vi "SeqListBox_EditMode.vi"(8 "error in (no error)":errorcluster, 10 "Debug":bool, 11 "GUI_Handler_Seq in":refnum<class "GUI_Handler_Seq.lvclass">) -> (0 "error out":errorcluster, 3 "GUI_Handler_Seq out":refnum<class "GUI_Handler_Seq.lvclass">)   [LabVIEW 2019, in "GUI_Handler_Seq.lvclass"]
uses:
  GUI_Handler_Seq.lvclass
panel:
  out "Size:Width":u32
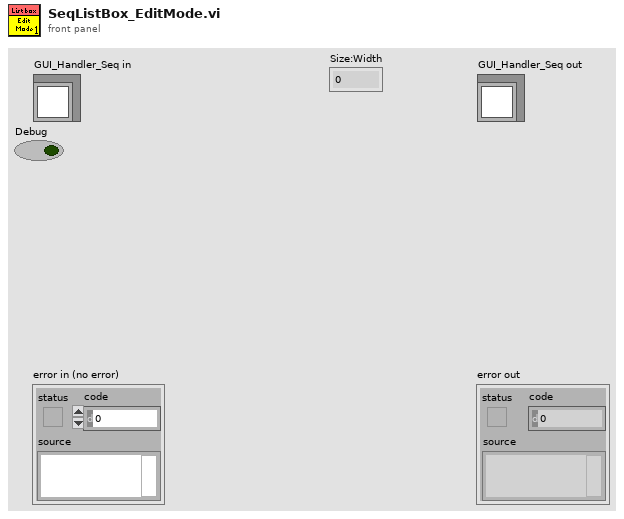
[diagram p1: front panel]
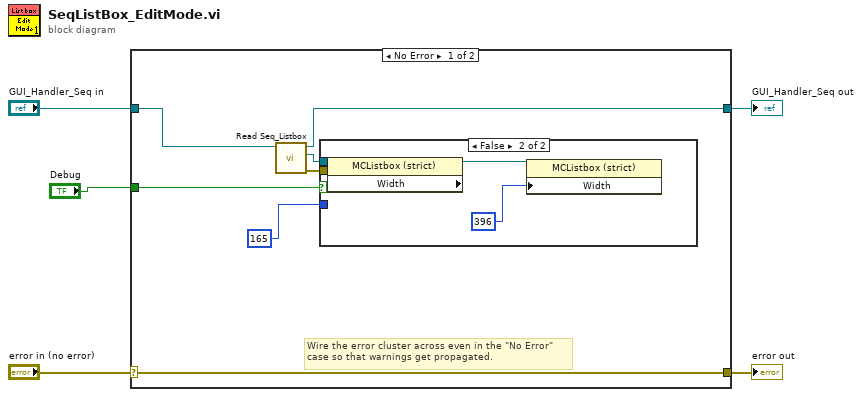
[diagram p0: block diagram]
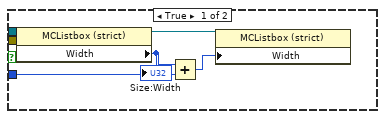
[diagram p2: hidden frame]
diagram:
  n1 = case shown="No Error" "error in (no error)" {
    selector: "error in (no error)" -> [w12 w24]
    tunnel: [w12 w24] -> w4
    tunnel: [w8 w23] -> w2
    tunnel: "GUI_Handler_Seq in" -> [w11 w23]
    tunnel: "Debug" -> [w7 _]
    frame No Error {
      # "Wire the error cluster across even in the \"No Error\"\ncase so that warnings get propagated."
      n2 = call-dynamic "Read Seq_Listbox.vi"("GUI_Handler_Seq in"=w11) -> ("error out"=w9:errorcluster, "Seq_Listbox"=w10:refnum<vi>, "GUI_Handler_Seq out"=w8:refnum<class "GUI_Handler_Seq.lvclass">)  [unwired: 8 in]
      n3 = case shown="False" w7 {
        tunnel: w10 -> [w18 w22]
        tunnel: w9 -> [w17 w21]
        tunnel: u32 165 ("y") -> [w13 _]
        frame True {
          n4 = property class="MCListbox (strict)"(reference=w18, error in=w17) -> (reference out=w14:refnum<vi>, "Width"=w15:u32)  [unwired: 1 out]
          "Size:Width" <- w15
          n5 = Add(x=w15, y=w13) -> (x+y=w16:u32)
          n6 = property class="MCListbox (strict)"(reference=w14, "Width"=w16) -> ()  [unwired: 1 in, 2 out]
        }
        frame False {
          n7 = property class="MCListbox (strict)" props=["Width"](reference=w22, error in=w21) -> (reference out=w20:refnum<vi>)  [unwired: 2 out]
          n8 = property class="MCListbox (strict)"(reference=w20, "Width"=u32 396 ("Size:Width")) -> ()  [unwired: 1 in, 2 out]
        }
      }
    }
    frame Error {
    }
  }
  "error out" <- w4
  "GUI_Handler_Seq out" <- w2
